vi "Set discriminator slope.vi"(8 "error in (no error)":errorcluster, 9 "j (0)":enum16{"Rise", "Fall"}(ring), 10 "i (0)":T1, 11 "VISA resource name":refnum<visa-resource-name>) -> (0 "error out":errorcluster, 3 "VISA resource name out":refnum<visa-resource-name>)   [LabVIEW 2015, in "SR400.lvlib"]
doc: "DS i { ,j }\nThe DS command sets and reads the discriminator\nslopes. i = 0,1, or 2 designates discriminator A,B,\nor T and is required. If j is included, the selected\ndiscriminator slope is set to RISE, j=0, or FALL,\nj=1. If j is absent, the slope of discriminator i is\nreturned."
uses:
  SR400.lvlib
  Typedefs/Counter.ctl
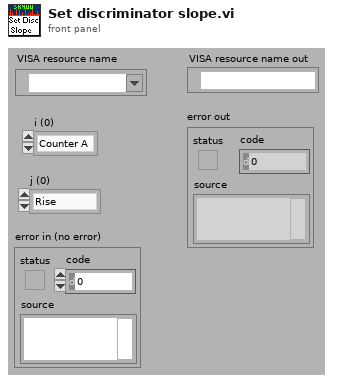
[diagram p1: front panel]
types:
  T1 = typedef "SR400.lvlib/Counter.ctl" = enum16{"Counter A", "Counter B", "Counter T"}
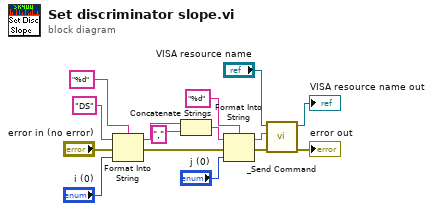
[diagram p0: block diagram]
diagram:
  n1 = Format Into String(format string="%d", initial string="DS" ("command"), error in="error in (no error)", "i (0)") -> (resulting string=w12:string, error out=w13:errorcluster)
  n2 = Concatenate Strings(w12, "," ("command")) -> (w7:string)
  n3 = Format Into String(format string="%d", initial string=w7, error in=w13, "j (0)") -> (resulting string=w4:string, error out=w3:errorcluster)
  n4 = call "_Send Command.vi"("error in (no error)"=w3, "Command"=w4, "VISA resource name"="VISA resource name") -> ("error out"=→"error out":errorcluster, "VISA resource name out"=→"VISA resource name out":refnum<visa-resource-name>)  [unwired: 1 in, 6 out]
